vi "RSZVB Start IMOD Receiver Power Calibration.vi"(8 "error in (no error)":errorcluster {"code" format="%.0x"}, 9 "Port (1)":i32=1, 10 "Channel (1)":i32=1, 11 "VISA session":refnum<visa-resource-name>) -> (0 "error out":errorcluster {"code" format="%.0x"}, 3 "dup VISA session":refnum<visa-resource-name>)   [LabVIEW 2011]
doc: "This VI starts the receiver calibration (2nd power calibration step for intermodulation measurements), stores and applies the calibration data. \n\nNote(s):\n\n(1) The receiver calibration relies on the source power calibration acquired in step no. 1. Use this VI after using rszvb_StartIMODLowerToneSourcePowerCalibration and rszvb_StartIMODUpperToneSourcePowerCalibration VIs.\n\n(2) This VI is not available for R&S ZVB instrument.\n\nRemote-control command(s):\n[SENSe<Ch>:]CORRection:POWer<port_no>:IMODulation:ACQuire"
uses:
  _utility/RSZVB Global Data.vi
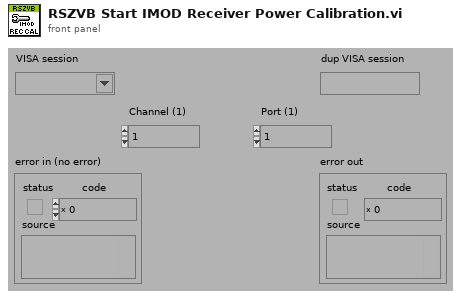
[diagram p1: front panel]
types:
  T1 = cluster{"Error Checking (T: On)":bool, "Installed Options":string[], "Data Valid?":bool, "Ports":i32, "Model":string[], "Option Checking (T: On)":bool}[]
  T2 = cluster{"Error Checking (T: On)":bool, "Installed Options":string[], "Data Valid?":bool, "Ports":i32, "Model":string[], "Option Checking (T: On)":bool}
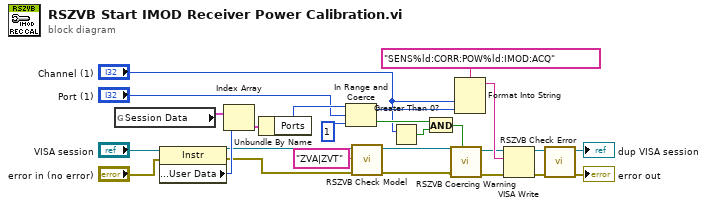
[diagram p0: block diagram]
diagram:
  n1 = global read "RSZVB Global Data.vi" "Session Data"() -> (w19:T1)
  n2 = property class="Instr"(reference="VISA session", error in="error in (no error)") -> (reference out=w2:refnum<visa-resource-name>, error out=w1:errorcluster, "General Settings:User Data"=w17:u32)
  n3 = Index Array(array=w19, index=w17) -> (element=w20:T2)
  n4 = Unbundle By Name(w20) -> ("Ports"=w16:i32)
  n5 = In Range and Coerce(upper limit=w16, x="Port (1)", lower limit=1) -> (coerced(x)=w15:i32, In Range?=w12:bool)
  n6 = call "RSZVB Check Model.vi"("error in (no error)"=w1, "Model"="ZVA|ZVT", "VISA session"=w2) -> ("error out"=w3:errorcluster, "dup VISA session"=w4:refnum<visa-resource-name>)  [unwired: 7 in]
  n7 = Greater Than 0?(x="Channel (1)") -> (x > 0?=w13:bool)
  n8 = And(x=w12, y=w13) -> (x .and. y?=w14:bool)
  n9 = call "RSZVB Coercing Warning.vi"("In Range?"=w14, "error in (no error)"=w3, "VISA session"=w4) -> ("error out"=w23:errorcluster, "dup VISA session"=w22:refnum<visa-resource-name>)  [unwired: 7 in]
  n10 = Format Into String(format string="SENS%ld:CORR:POW%ld:IMOD:ACQ", "Channel (1)", w15) -> (resulting string=w24:string)  [unwired: 2 in, 1 out]
  n11 = VISA Write(VISA resource name=w22, write buffer=w24, error in (no error)=w23) -> (VISA resource name out=w25:refnum<visa-resource-name>, error out=w26:errorcluster)  [unwired: 1 out]
  n12 = call "RSZVB Check Error.vi"("error in (no error)"=w26, "VISA session"=w25) -> ("error out"=→"error out":errorcluster, "dup VISA session"=→"dup VISA session":refnum<visa-resource-name>)  [unwired: 8 in]
